vi "Remove Session Info to Unreserve.vi"(8 "error in":errorcluster, 10 "session reservation":refnum<class "Session Reservation.lvclass">, 11 "measurement context in":refnum<class "MeasurementContext.lvclass">) -> (0 "error out":errorcluster, 3 "measurement context out":refnum<class "MeasurementContext.lvclass">)   [LabVIEW 2020, in "MeasurementLink Measurement Server.lvlib" / "MeasurementContext.lvclass"]
uses:
  MeasurementContext.lvclass
  MeasurementContext.lvclass/MeasurementContext.ctl
  MeasurementLink Session Management/Session Reservation/Session Reservation.lvclass
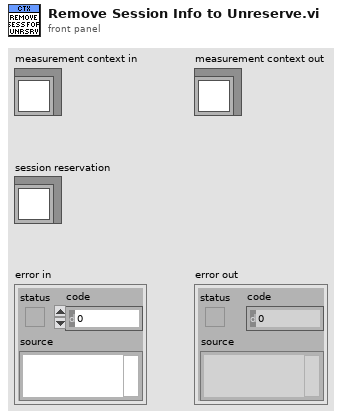
[diagram p1: front panel]
types:
  T1 = typedef "MeasurementLink Measurement Server.lvlib/MeasurementContext.lvclass/Data.ctl" = cluster{"PinMapContext":T2, "gRPCServerId":T3, "IMeasurementService":refnum<class "IMeasurementService.lvclass">, "MeasurementPluginService":refnum<class "MeasurementPluginService.lvclass">, "session infos to unreserve":map{refnum<class "Session Reservation.lvclass">, T4[]}}
  T2 = typedef "MeasurementLink Measurement Server.lvlib/PinMapContext.ctl" = cluster{"pin_map_id":string, "sites":i32[]}
  T3 = typedef "grpc-lvsupport-release.lvlib/grpcId.ctl" = u64
  T4 = typedef "MeasurementLink Session Management Client.lvlib/ni_measurementlink_sessionmanagement_v1_SessionInformation.ctl" = cluster{"session":T5, "resource_name":string, "channel_list":string, "instrument_type_id":string, "session_exists":bool, "channel_mappings":T6[]}
  T5 = typedef "MeasurementLink Session Management Client.lvlib/nidevice_grpc_Session.ctl" = cluster{"name":string}
  T6 = typedef "MeasurementLink Session Management Client.lvlib/ni_measurementlink_sessionmanagement_v1_ChannelMapping.ctl" = cluster{"pin_or_relay_name":string, "site":i32, "channel":string}
  T7 = map{refnum<class "Session Reservation.lvclass">, T4[]}
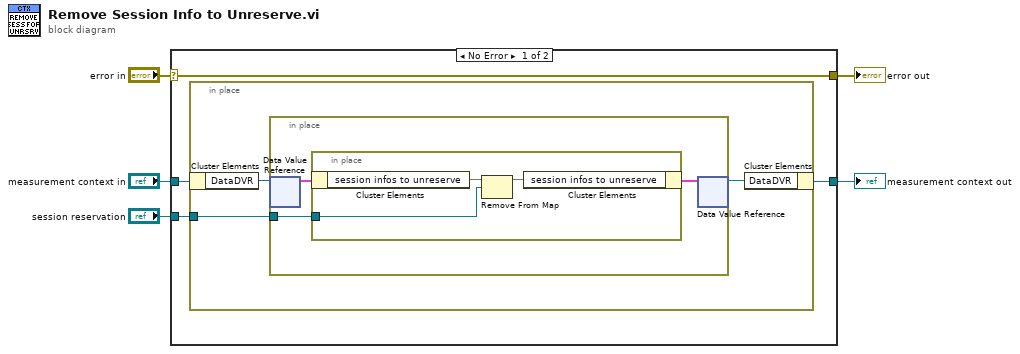
[diagram p0: block diagram]
diagram:
  n1 = case shown="No Error" "error in" {
    selector: "error in" -> [w8 w20]
    tunnel: [w8 w20] -> w4
    tunnel: [w7 w19] -> w2
    tunnel: "measurement context in" -> [w9 w19]
    tunnel: "session reservation" -> [w6 _]
    frame No Error {
      n2 = in-place {
        in-place-border: w6 -> [w10]
        n3 = in-place-cluster #1(w9) -> ("DataDVR"=w12:refnum<data-value>)
        n4 = in-place {
          in-place-border: w10 -> [w13]
          n5 = in-place-dvr #2(w12) -> (w15:T1)  [unwired: 1 out]
          n6 = in-place {
            in-place-border: w13 -> [w17]
            n7 = in-place-cluster #3(w15) -> ("session infos to unreserve"=w18:T7)
            n8 = Remove From Map(10:w17, 11:w18) -> (3:w16:T7)  [unwired: 2 out]
            n9 = in-place-cluster #3("session infos to unreserve"=w16) -> (w14:T1)
          }
          n10 = in-place-dvr #2(w14) -> (w11:refnum<data-value>)  [unwired: 1 out]
        }
        n11 = in-place-cluster #1("DataDVR"=w11) -> (w7:refnum<class "MeasurementContext.lvclass">)
      }
    }
    frame Error {
    }
  }
  "error out" <- w4
  "measurement context out" <- w2
